vi "String_parsingV6.vi"(9 "input string":string) -> (0 "hour":i32, 1 "V2":i32[](array[numeric]), 2 "V3":i32[](array[numeric]), 3 "V1":i32[](array[numeric]), 5 "timeStamp_ms":i32[](array[numeric]), 6 "minute":i32, 7 "sekundes":i32, 8 "size(s)":i32)   [LabVIEW 2014]
panel:
  out "input test":u8[](array[numeric])
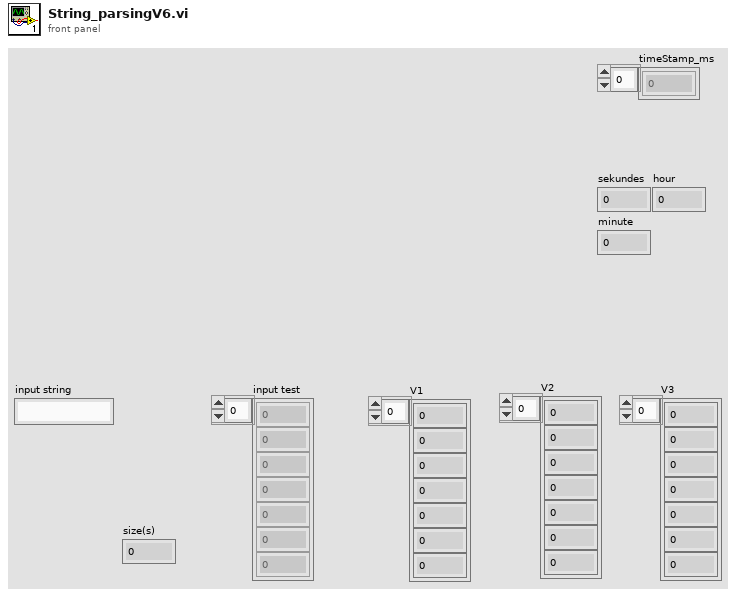
[diagram p1: front panel]
types:
  T1 = typedef "LVDateTimeRec.ctl" = cluster{"fractional second":dbl, "second":i32, "minute":i32, "hour":i32, "day of month":i32, "month":i32, "year":i32, "day of week":i32, "day of year":i32, "DST":i32}
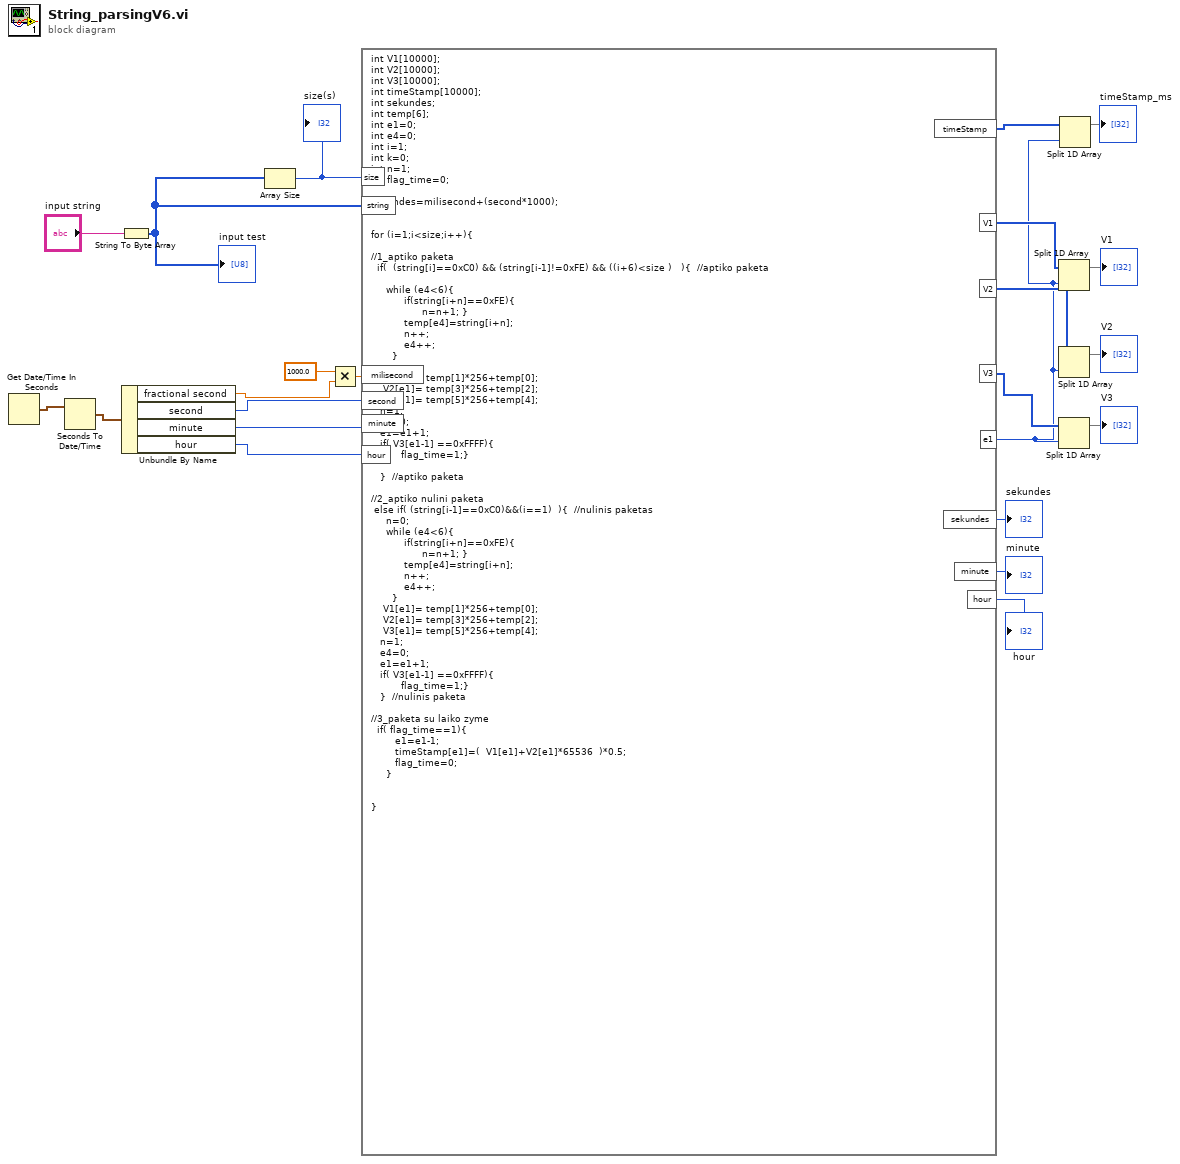
[diagram p0: block diagram]
diagram:
  n1 = Get Date/Time In Seconds() -> (seconds since 1Jan1904=w14:timestamp)
  n2 = Seconds To Date/Time(time stamp (now)=w14) -> (date time rec=w13:T1)  [unwired: 1 in]
  n3 = String To Byte Array(string="input string") -> (unsigned byte array=w23:u8[])
  "input test" <- w23
  n4 = Unbundle By Name(w13) -> ("fractional second"=w9:dbl, "second"=w12:i32, "minute"=w11:i32, "hour"=w10:i32)
  n5 = Array Size(array=w23) -> (size(s)=w22:i32)
  "size(s)" <- w22
  n6 = Multiply(x=1000.0, y=w9) -> (x*y=w7:dbl)
  n7 = formula code="int V1[10000];\nint V2[10000];\nint V3[10000];\nint timeStamp[10000];\nint sekundes;\nint temp[6];\nint e1=0;\nint e4=0;\nint i=1;\nint k=0;\nint n=1;\nint flag_time=0;\n\nsekundes=milisecond+(second*1000);\n\n\nfor (i=1;i<size;i++){\n \n//1_aptiko paketa\n  if(  (string[i]==0xC0) && (string[i-1]!=0xFE) && ((i+6)<size )   ){  //aptiko paketa\n\n     while (e4<6){\n           if(string[i+n]==0xFE){\n                 n=n+1; }\n           temp[e4]=string[i+n];\n           n++; \n           e4++;\n       }\n   \n    V1[e1]= temp[1]*256+temp[0];\n    V2[e1]= temp[3]*256+temp[2];\n    V3[e1]= temp[5]*256+temp[4];\n   n=1;\n   e4=0;\n   e1=e1+1;\n   if( V3[e1-1] ==0xFFFF){\n          flag_time=1;}\n   \n   }  //aptiko paketa\n\n//2_aptiko nulini paketa\n else if( (string[i-1]==0xC0)&&(i==1)  ){  //nulinis paketas\n     n=0;\n     while (e4<6){\n           if(string[i+n]==0xFE){\n                 n=n+1; }\n           temp[e4]=string[i+n];\n           n++; \n           e4++;\n       }\n    V1[e1]= temp[1]*256+temp[0];\n    V2[e1]= temp[3]*256+temp[2];\n    V3[e1]= temp[5]*256+temp[4];\n   n=1;\n   e4=0;\n   e1=e1+1;\n   if( V3[e1-1] ==0xFFFF){\n          flag_time=1;}\n   }  //nulinis paketa\n\n//3_paketa su laiko zyme\n  if( flag_time==1){\n        e1=e1-1;\n        timeStamp[e1]=(  V1[e1]+V2[e1]*65536  )*0.5; \n        flag_time=0;\n     }\n\n\n}"("string"=w23, "size"=w22, "milisecond"=w7, "second"=w12, "minute"=w11, "hour"=w10) -> ("V1"=w20:i32[], "V2"=w16:i32[], "V3"=w15:i32[], "e1"=w2:i32, "sekundes"=→"sekundes":i32, "minute"=→"minute":i32, "hour"=→"hour":i32, "timeStamp"=w3:i32[])
  n8 = Split 1D Array(array=w20, index=w2) -> (first subarray=→"V1":i32[])  [unwired: 1 out]
  n9 = Split 1D Array(array=w16, index=w2) -> (first subarray=→"V2":i32[])  [unwired: 1 out]
  n10 = Split 1D Array(array=w15, index=w2) -> (first subarray=→"V3":i32[])  [unwired: 1 out]
  n11 = Split 1D Array(array=w3, index=w2) -> (first subarray=→"timeStamp_ms":i32[])  [unwired: 1 out]
